vi "Read Fluid Name.vi"(8 "error in (no error)":errorcluster, 10 "Node (3)":u8=3 caption="Node" min=3 max=128 step=1, 11 "VISA resource name":refnum<visa-resource-name>) -> (0 "error out":errorcluster, 2 "Fluid Name":string, 3 "VISA resource name out":refnum<visa-resource-name>)   [LabVIEW 2019, in "Bronkhorst FLOW-BUS.lvlib"]
doc: "Reads the fluid name. Up to 10 characters are available for storage of this name. This parameter is secured and read only for normal users (it is written during calibration at the factory). Default value is \"Air\"."
uses:
  Bronkhorst FLOW-BUS.lvlib
  Private/FLOW-BUS RW.ctl
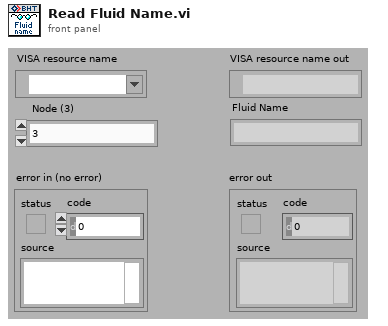
[diagram p1: front panel]
types:
  T1 = typedef "Bronkhorst FLOW-BUS.lvlib/FLOW-BUS RW.ctl" = cluster{"Node Address (3)":u8, "Communication Command":enum16{"Status message", "Send parameter with destination address and 00 response", "Send parameter with destination address", "Request parameter"}, "Process (0)":u16, "Parameter (0)":u16, "Data Type (0: Character)":enum16{"Character", "Integer", "Float or Long", "String"}, "Data for Char or Int (0)":u32, "Data for Float or Long (0)":sgl, "Data for String":string, "Length of Requested String (0)":u8}
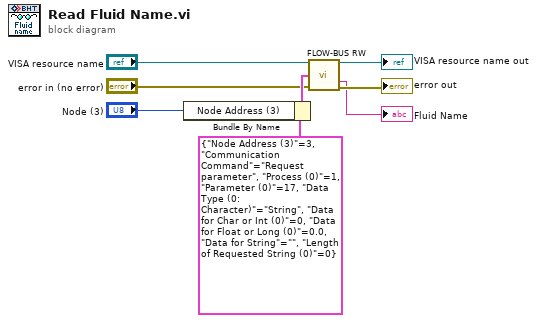
[diagram p0: block diagram]
diagram:
  n1 = Bundle By Name(cluster=T1 {"Node Address (3)"=3, "Communication Command"=enum."Request parameter", "Process (0)"=1, "Parameter (0)"=17, "Data Type (0: Character)"=enum."String", "Data for Char or Int (0)"=0, "Data for Float or Long (0)"=0.0, "Data for String"="", "Length of Requested String (0)"=0} ("FLOW-BUS Command Settings"), "Node Address (3)"="Node (3)") -> (w8:T1)
  n2 = call "FLOW-BUS RW.vi"("VISA resource name"="VISA resource name", "FLOW-BUS Command Settings"=w8, "error in (no error)"="error in (no error)") -> ("VISA resource name out"=→"VISA resource name out":refnum<visa-resource-name>, "Requested String"=→"Fluid Name":string, "error out"=→"error out":errorcluster)  [unwired: 8 in, 2 out]
